vi "Read AO_index.vi"(11 "bronkhorst_reg in":refnum<class "bronkhorst_reg_2.lvclass">) -> (2 "AO_index":i32, 3 "bronkhorst_reg out":refnum<class "bronkhorst_reg_2.lvclass">)   [LabVIEW 2019, in "control.lvlib" / "bronkhorst_reg_2.lvclass"]
uses:
  bronkhorst_reg_2.lvclass
  bronkhorst_reg_2.lvclass/bronkhorst_reg_2.ctl
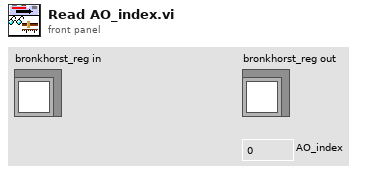
[diagram p1: front panel]
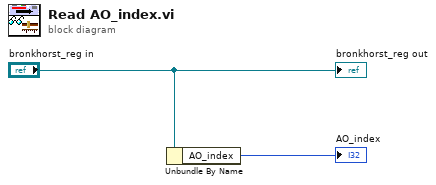
[diagram p0: block diagram]
diagram:
  n1 = Unbundle By Name("bronkhorst_reg in") -> ("AO_index"=→"AO_index":i32)
  "bronkhorst_reg out" <- "bronkhorst_reg in"
